vi "RM.forceAddReservation.vi"(7 "Resource Type":T1, 8 "error in":errorcluster, 9 "clientGUID":string, 10 "name in bitfile":string, 11 "reservation DB in":variant) -> (0 "error out":errorcluster, 1 "replaced":bool, 3 "reservation DB out":variant)   [LabVIEW 2016, in "FPGA Resource Manager.lvlib"]
uses:
  FPGA Resource Manager.lvlib
  RM.resourceType.ctl
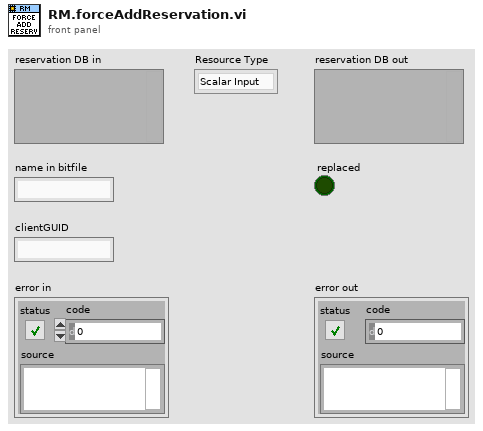
[diagram p1: front panel]
types:
  T1 = typedef "FPGA Resource Manager.lvlib/RM.resourceType.ctl" = enum16{"Scalar Input", "Scalar Output", "Waveform Input", "Waveform Output"}
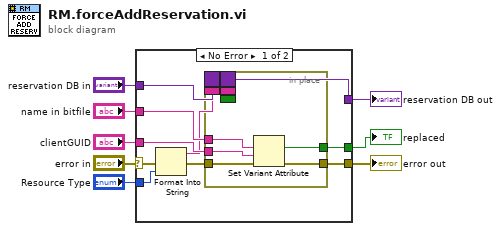
[diagram p0: block diagram]
diagram:
  n1 = case shown="No Error" "error in" {
    selector: "error in" -> [w11 w26]
    tunnel: "reservation DB in" -> [w18 w27]
    tunnel: [w17 w27] -> w7
    tunnel: "name in bitfile" -> [w16 _]
    tunnel: "clientGUID" -> [w15 _]
    tunnel: "Resource Type" -> [w14 _]
    tunnel: [w10 w26] -> w2
    tunnel: [w9 _] -> w1
    frame No Error {
      n2 = Format Into String(error in=w11, w14) -> (resulting string=w13:string, error out=w12:errorcluster)  [unwired: 2 in]
      n3 = in-place {
        border: w18 -> [_]
        border: w13 -> [_]
        border: [_] -> w17
        border: _ -> [_]
        border: _ -> [_]
        in-place-border: w16 -> [w25]
        in-place-border: w15 -> [w24]
        in-place-border: w12 -> [w23]
        in-place-border: [w22] -> w10
        in-place-border: [w21] -> w9
        n4 = Set Variant Attribute(Variant=w20, name=w25, value=w24, error in=w23) -> (Variant out=w19:variant, replaced=w21:bool, error out=w22:errorcluster)
      }
    }
    frame Error {
    }
  }
  "reservation DB out" <- w7
  "error out" <- w2
  "replaced" <- w1
